vi "NO MFR loff.vi"(8 "Flow Rate":dbl, 9 "NO Measured ppm":dbl, 10 "NO Conc":dbl, 11 "NOx Target ppm":dbl) -> (2 "NO MFR":dbl)   [LabVIEW 2011]
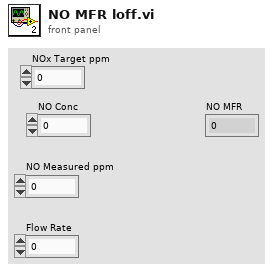
[diagram p1: front panel]
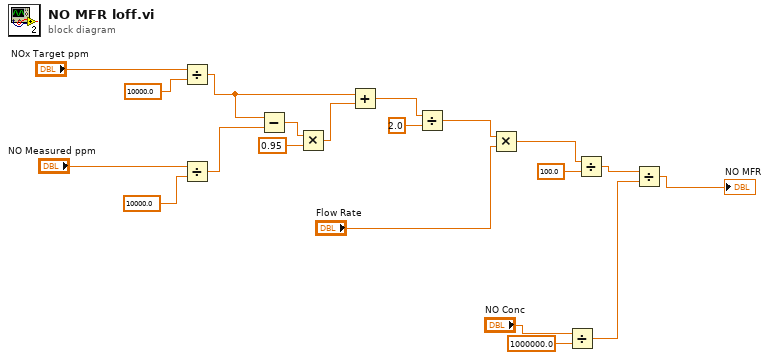
[diagram p0: block diagram]
diagram:
  n1 = Divide(x="NOx Target ppm", y=10000.0) -> (x/y=w8:dbl)
  n2 = Divide(x="NO Measured ppm", y=10000.0) -> (x/y=w9:dbl)
  n3 = Subtract(x=w8, y=w9) -> (x-y=w7:dbl)
  n4 = Multiply(x=w7, y=0.95) -> (x*y=w6:dbl)
  n5 = Add(x=w8, y=w6) -> (x+y=w1:dbl)
  n6 = Divide(x=w1, y=2.0) -> (x/y=w2:dbl)
  n7 = Multiply(x=w2, y="Flow Rate") -> (x*y=w15:dbl)
  n8 = Divide(x="NO Conc", y=1000000.0) -> (x/y=w10:dbl)
  n9 = Divide(x=w15, y=100.0) -> (x/y=w14:dbl)
  n10 = Divide(x=w14, y=w10) -> (x/y=→"NO MFR":dbl)
